vi "Main.vi"(9 "rSubPanel":refnum<vi>, 10 "模块定义":T1, 11 "Module Admin":refnum<class "Delacor_lib_QMH_Cloneable Module Admin.lvclass">) -> ()   [LabVIEW 2018, in "ModuleInterface.lvlib"]
doc: "This template is based off of the Queued Message Handler design pattern and the Queued Message Handler project template that ships with LabVIEW.\n\nThe main difference is that the queue is private to this module and communication between modules is performed via Broadcast and Request events.\n\nRequest events are wrapped in public API methods and are handled in the Event Handling Loop (EHL) of this VI. Any module can register for Broadcast events sent by this module. The EHL generates messages based on user interface actions.\n\nThe Message Handling Loop (MHL) processes messages generated by the EHL, or by other messages. The messages are string values, so new messages can be added easily to the Message Cases case structure in the MHL. Each message cluster can also provide an optional value for Message Data, which is a variant that can be converted to whatever message-specific data is required.\n_____\nBased on DQMH Project Template 7.0.1.1316."
uses:
  ModuleInterface.lvlib
  <vilib>/Delacor/Delacor QMH/Libraries/Cloneable Module Admin_class/Delacor_lib_QMH_Cloneable Module Admin.lvclass
  C:/Program Files (x86)/National Instruments/LabVIEW 2018/vi.lib/Delacor/Delacor QMH/Libraries/Module Admin_class/Delacor_lib_QMH_Module Admin.lvclass
  Buttons/FoldButton.ctl
  ModuleDefinition.ctl
  FunctionItem.ctl
  Module Data--cluster.ctl
  <vilib>/Delacor/Delacor QMH/Libraries/Message Queue_class/Delacor_lib_QMH_Message Queue.lvclass/Delacor_lib_QMH_Message Queue.ctl
  <vilib>/Delacor/Delacor QMH/Libraries/Cloneable Module Admin_class/Delacor_lib_QMH_Cloneable Module Admin.lvclass/Delacor_lib_QMH_Cloneable Module Admin.ctl
  Stop Argument--cluster.ctl
  <vilib>/Delacor/Delacor QMH/Libraries/Module Admin_class/Delacor_lib_QMH_Module Admin.lvclass/Delacor_lib_QMH_Module Admin.ctl
  Get Module Name Argument--cluster.ctl
  Get Module Name (Reply Payload)--cluster.ctl
  Get Module ID List Argument--cluster.ctl
  Get Module ID List (Reply Payload)--cluster.ctl
  Disable Item Argument--cluster.ctl
  Enable Item Argument--cluster.ctl
  <vilib>/Utility/miscctls.llb/LVPointTypeDef.ctl
  Clone Registration/Action--enum.ctl
  <vilib>/Delacor/Delacor QMH/Libraries/Message Queue_class/Delacor_lib_QMH_Enqueue Message (Single).vi
  <vilib>/Delacor/Delacor QMH/Libraries/Cloneable Module Admin_class/Delacor_lib_QMH_Get Module ID.vi
  <vilib>/Delacor/Delacor QMH/Libraries/Module Admin_class/Delacor_lib_QMH_Get External Launch.vi
  <vilib>/Delacor/Delacor QMH/Libraries/Message Queue_class/Delacor_lib_QMH_Message Queue.lvclass
  Clone Registration/Clone Registration.lvlib
panel:
  in  "界面单元":T4={"ModuleName"="", "FunctionList"=0, "展收按钮"=TRUE, "Spacer"=""}
  out "error out":errorcluster
  out "Status":string
  in  "Simulate EHL Error":bool
  in  "Simulate MHL Error":bool
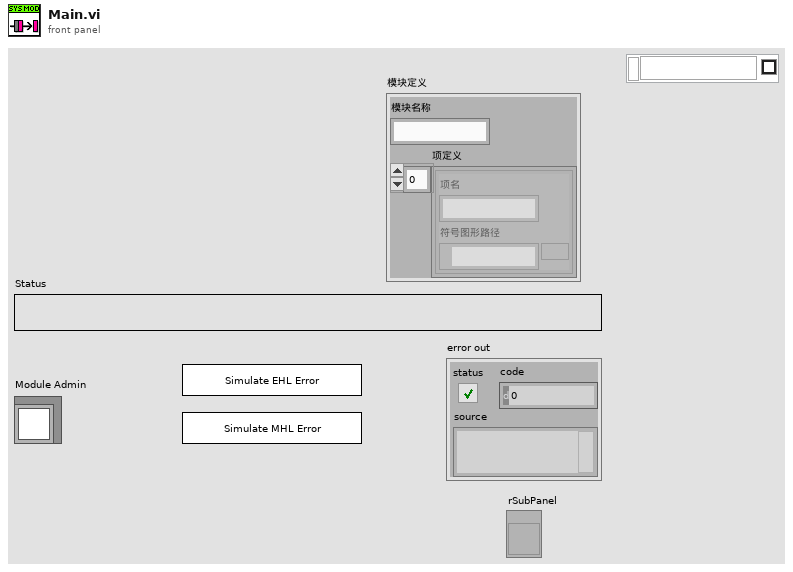
[diagram p1: front panel]
types:
  T1 = typedef "ModuleInterface.lvlib/ModuleDefinition.ctl" = cluster{"模块名称":string, "项定义":T2[]}
  T2 = typedef "ModuleInterface.lvlib/FunctionItem.ctl" = cluster{"项名":string, "符号图形路径":path}
  T3 = typedef "FoldButton.ctl" = bool
  T4 = cluster{"ModuleName":string, "FunctionList":i32, "展收按钮":T3, "Spacer":string}
  T5 = typedef "ModuleInterface.lvlib/Request Events--cluster.ctl" = cluster{"Stop Module":refnum<user-event>, "Show Panel":refnum<user-event>, "Hide Panel":refnum<user-event>, "Show Diagram":refnum<user-event>, "Get Module Execution Status":refnum<user-event>, "Get Module Name":refnum<user-event>, "Get Module ID List":refnum<user-event>, "Disable Item":refnum<user-event>, "Enable Item":refnum<user-event>}
  T6 = typedef "ModuleInterface.lvlib/Module Data--cluster.ctl" = cluster{"Status":string, "rSubPanel":refnum<vi>, "Disabled Items":string[]}
  T7 = enum32{"invalid lock state", "Not Locked", "Locked (No Password)", "Password-protected"}
  T8 = typedef "ModuleInterface.lvlib/Stop Argument--cluster.ctl" = cluster{"Module ID":i32, "Origin":string, "Exit via Stop Module Req?":bool, "Wait for Module to stop?":bool}
  T9 = typedef "ModuleInterface.lvlib/Get Module Name Argument--cluster.ctl" = cluster{"Module ID":i32, "Wait Notifier":refnum<notifier>, "wait for reply":bool}
  T10 = typedef "ModuleInterface.lvlib/Get Module ID List Argument--cluster.ctl" = cluster{"Module ID":i32, "Wait Notifier":refnum<notifier>, "wait for reply":bool}
  T11 = typedef "ModuleInterface.lvlib/Disable Item Argument--cluster.ctl" = cluster{"Module ID":i32, "Item Name":string}
  T12 = typedef "ModuleInterface.lvlib/Enable Item Argument--cluster.ctl" = cluster{"Module ID":i32, "Item Name":string}
  T13 = enum32{"Invalid", "Standard", "Closed", "Hidden", "Minimized", "Maximized"}
  T14 = typedef "LVPointTypeDef.ctl" = cluster{"Horizontal":i16, "Vertical":i16}
  T15 = typedef "ModuleInterface.lvlib/Get Module Name (Reply Payload)--cluster.ctl" = cluster{"Module ID":i32, "Module Name":string, "error":errorcluster}
  T16 = typedef "ModuleInterface.lvlib/Clone Registration.lvlib/Action--enum.ctl" = enum16{"Init", "Add Instance", "Remove Instance", "List Instances", "Is First?"}
  T17 = typedef "ModuleInterface.lvlib/Get Module ID List (Reply Payload)--cluster.ctl" = cluster{"Module ID":i32, "Module ID List":i32[], "error":errorcluster}
  T18 = typedef "LVRectTypeDef.ctl" = cluster{"Left":i16, "Top":i16, "Right":i16, "Bottom":i16}
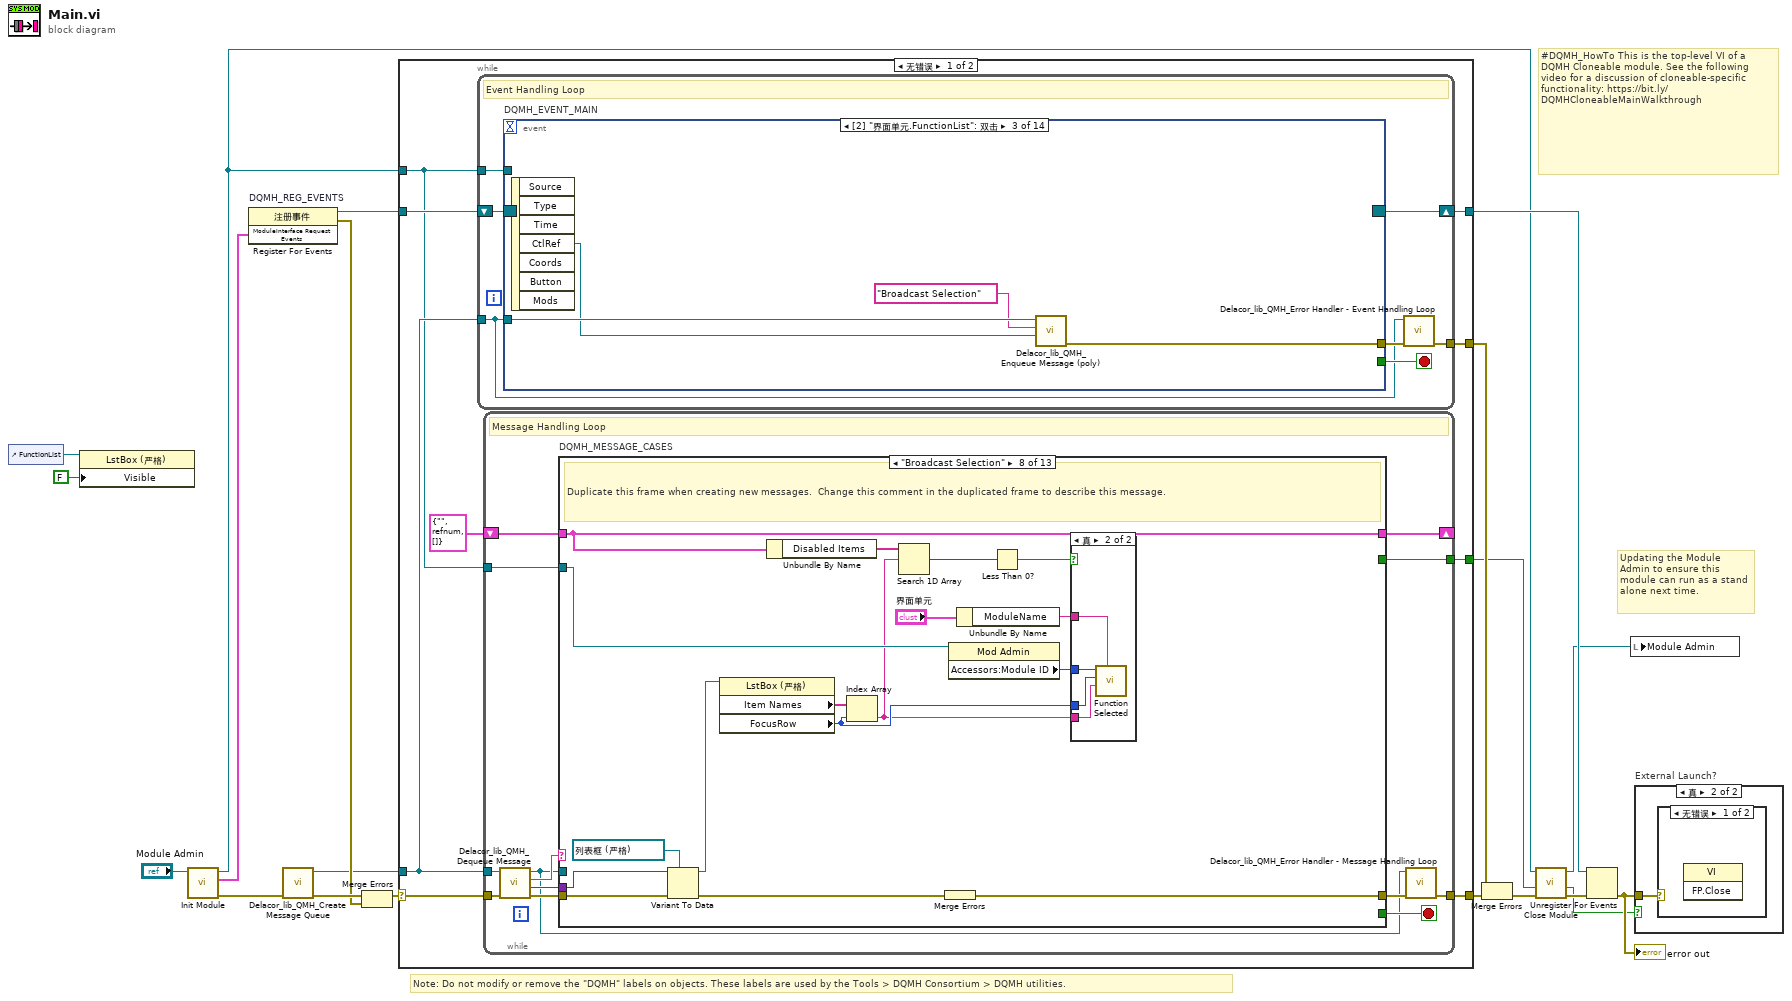
[diagram p0: block diagram]
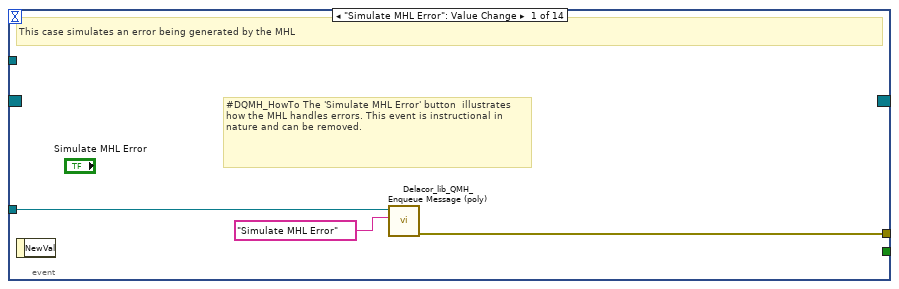
[diagram p2: hidden frame]
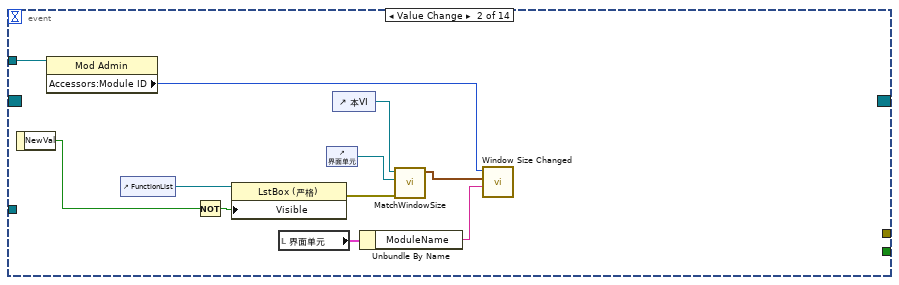
[diagram p3: hidden frame]
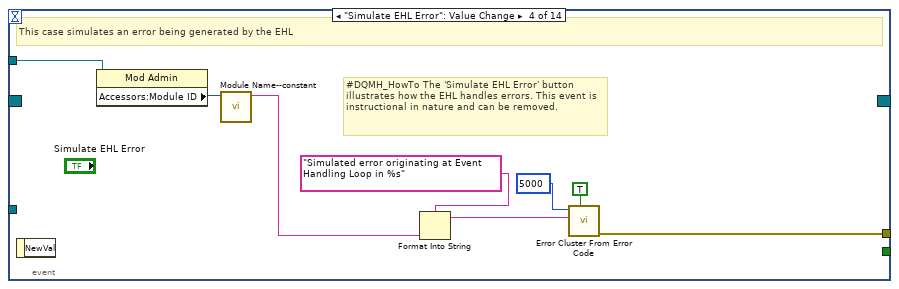
[diagram p4: hidden frame]
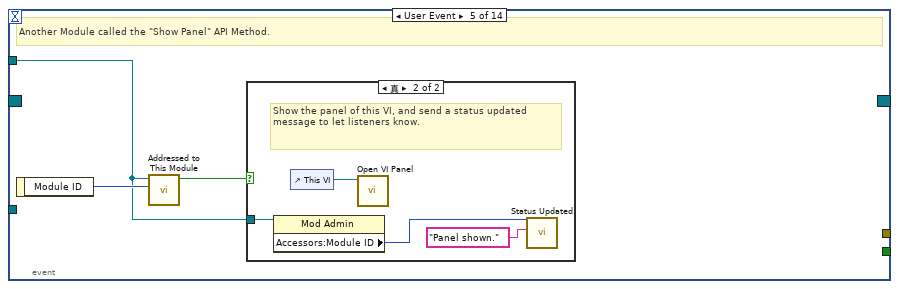
[diagram p5: hidden frame]
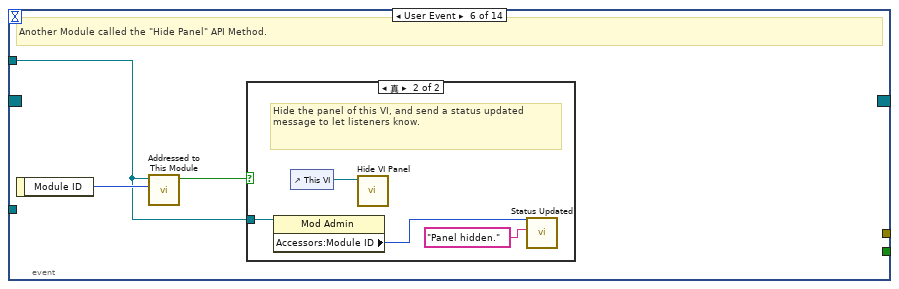
[diagram p7: hidden frame]
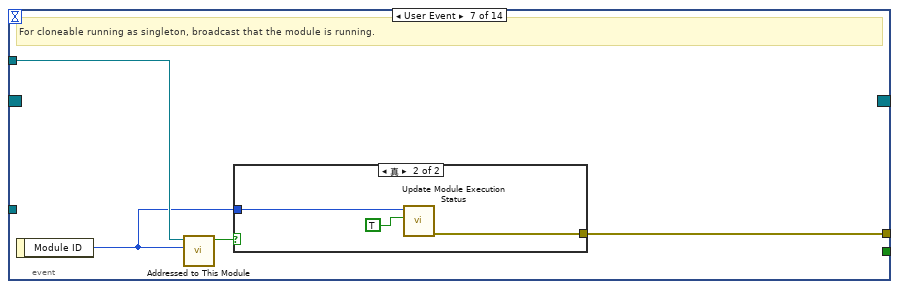
[diagram p9: hidden frame]
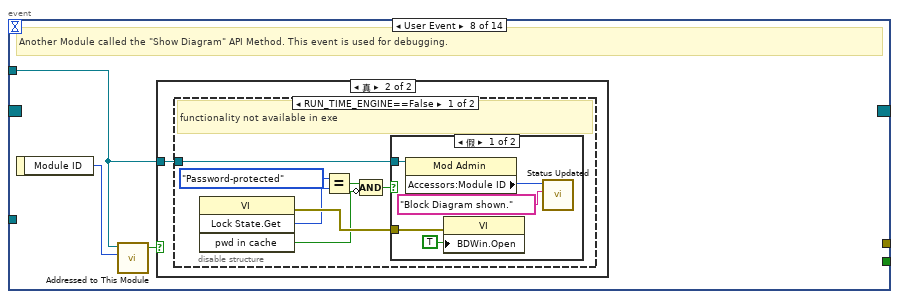
[diagram p11: hidden frame]
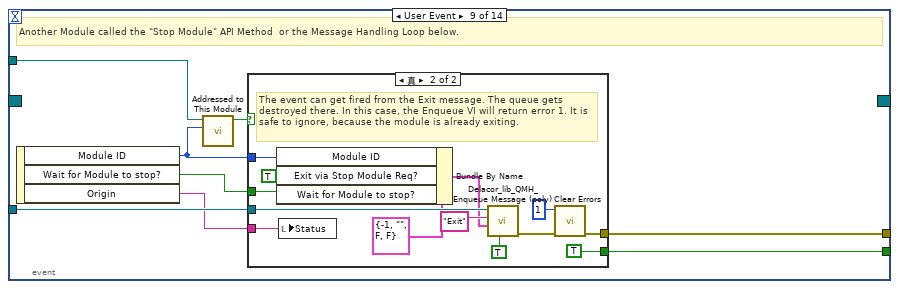
[diagram p15: hidden frame]
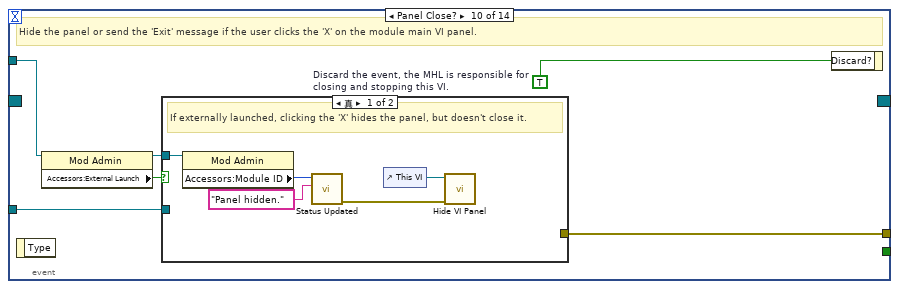
[diagram p17: hidden frame]
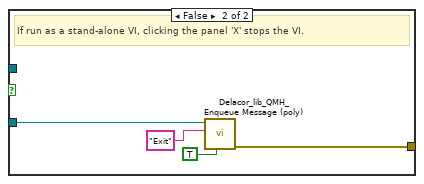
[diagram p18: hidden frame]
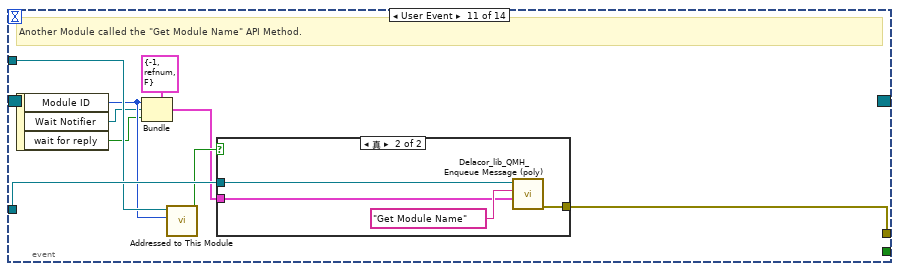
[diagram p19: hidden frame]
diagram:
  # "#DQMH_HowTo This is the top-level VI of a DQMH Cloneable module. See the following video for a discussion of cloneable-specific functionality: https://bit.ly/DQMHCloneableMainWalkthrough"
  # "Note: Do not modify or remove the \"DQMH\" labels on objects. These labels are used by the Tools > DQMH Consortium > DQMH utilities."
  # "Updating the Module Admin to ensure this module can run as a stand alone next time."
  n1 = control-ref of="FunctionList"() -> (w1:refnum<vi>)
  n2 = property class="LstBox (严格)"(reference=w1, "Visible"=FALSE ("可见")) -> ()  [unwired: 1 in, 2 out]
  n3 = call "Init Module.vi"("Cloneable Module Admin in"="Module Admin") -> ("error out"=w17:errorcluster, "ModuleInterface Request Events"=w9:T5, "Cloneable Module Admin out"=w6:refnum<class "Delacor_lib_QMH_Cloneable Module Admin.lvclass">)  [unwired: 8 in]
  n4 = register-events "DQMH_REG_EVENTS"(w9) -> (reference out=w10:refnum<event-registration>, error out=w12:errorcluster)  [unwired: 2 in]
  n5 = call <vilib>:"Delacor_lib_QMH_Create Message Queue.vi"("error in"=w17) -> ("error out"=w14:errorcluster, "Message Queue"=w8:refnum<class "Delacor_lib_QMH_Message Queue.lvclass">)  [unwired: 9 in]
  n6 = Merge Errors(w14, w12) -> (w13:errorcluster)
  n7 = case shown="无错误" w13 {
    selector: w13 -> [w27 w408]
    tunnel: [w29 w407] -> w18
    tunnel: [w26 w406] -> w11
    tunnel: w10 -> [w24 w406]
    tunnel: w8 -> [w23 w399]
    tunnel: [w28 _] -> w19
    tunnel: w6 -> [w22 w402]
    tunnel: [w21 _] -> w4
    frame No Error {
      n8 = while {
        tunnel: w23 -> [w30]
        shift-right: [w33] -> w26
        shift-left: w24 -> [w34]
        tunnel: [w35] -> w28
        tunnel: w22 -> [w31]
        stop <- w32 stop-if-true
        # "Event Handling Loop"
        n9 = event "DQMH_EVENT_MAIN" shown="[2] \"界面单元.FunctionList\": 双击" {
          selector: w34 -> [_ _ _ _ _ _ _ _ _ _ _ _ _ _]
          dyn-events: [_ _ _ _ _ _ _ _ _ _ _ _ _ _] -> w33
          timeout: _ -> [_ _ _ _ _ _ _ _ _ _ _ _ _ _]
          tunnel: [_ _ _ _ _ _ _ _ w103 _ _ _ _ _] -> w32
          tunnel: w30 -> [w38 _ w54 _ _ _ _ _ w106 w123 w144 w157 w169 w181]
          tunnel: [w39 _ w53 w62 _ _ w80 _ w107 w126 w136 w149 w162 w174] -> w36
          tunnel: w31 -> [_ w44 _ w61 w63 w70 w78 w84 w105 w124 w142 w155 w167 w179]
          event "Simulate MHL Error": Value Change {
            # "#DQMH_HowTo The 'Simulate MHL Error' button  illustrates how the MHL handles errors. This event is instructional in nature and can be removed."
            # "This case simulates an error being generated by the MHL"
            n10 = event-data() -> ()  [unwired: 1 in, 1 out]
            n11 = call-poly <vilib>:"Delacor_lib_QMH_Enqueue Message (poly).vi"("Message"="Simulate MHL Error", "Message Queue in"=w38) -> ("error out"=w39:errorcluster)  [unwired: 8 in, 1 out]
          }
          event Value Change {
            n12 = event-data() -> ("NewVal"=w49:T3)  [unwired: 1 in]
            n13 = property on="Property Node" class="Mod Admin"(reference=w44) -> ("Accessors:Module ID"=w42:i32)  [unwired: 1 in, 2 out]
            n14 = control-ref of="FunctionList"() -> (w50:refnum<vi>)
            n15 = Not(x=w49) -> (.not. x?=w48:T3)
            n16 = property class="LstBox (严格)"(reference=w50, "Visible"=w48) -> (error out=w46:errorcluster)  [unwired: 1 in, 1 out]
            n17 = local read "界面单元"() -> (w41:T4)
            n18 = control-ref of="界面单元"() -> (w47:refnum<vi>)
            n19 = control-ref of="本VI"() -> (w45:refnum<vi>)
            n20 = Unbundle By Name(w41) -> ("ModuleName"=w40:string)
            n21 = call "MatchWindowSize.vi"("错误输入（无错误）"=w46, "界面单元"=w47, "VI输入"=w45) -> ("窗口边界"=w43:T18)  [unwired: 7 in, 1 out]
            n22 = call "Window Size Changed.vi"("Module Name"=w40, "窗口边界"=w43, "Module ID"=w42) -> ()  [unwired: 8 in, 1 out]
          }
          event "界面单元.FunctionList": Double Click {
            n23 = event-data() -> ("CtlRef"=w52:refnum<vi>)  [unwired: 1 in, 6 out]
            n24 = call-poly <vilib>:"Delacor_lib_QMH_Enqueue Message (poly).vi"("Message Data"=w52, "Message"="Broadcast Selection", "Message Queue in"=w54) -> ("error out"=w53:errorcluster)  [unwired: 7 in, 1 out]
          }
          event "Simulate EHL Error": Value Change {
            # "#DQMH_HowTo The 'Simulate EHL Error' button  illustrates how the EHL handles errors. This event is instructional in nature and can be removed."
            # "This case simulates an error being generated by the EHL"
            n25 = event-data() -> ()  [unwired: 1 in, 1 out]
            n26 = property on="Property Node" class="Mod Admin"(reference=w61) -> ("Accessors:Module ID"=w60:i32)  [unwired: 1 in, 2 out]
            n27 = call "Module Name--constant.vi"("Module ID"=w60) -> ("Module Name"=w55:string)  [unwired: 10 in]
            n28 = Format Into String(format string="Simulated error originating at Event Handling Loop in %s", w55) -> (resulting string=w58:string)  [unwired: 2 in, 1 out]
            n29 = call <vilib>:"Error Cluster From Error Code.vi"("show call chain? (False)"=TRUE, "error message (\"\")"=w58, "error code (0)"=5000) -> ("error out"=w62:errorcluster)  [unwired: 6 in]
          }
          event User Event {
            # "Another Module called the \"Show Panel\" API Method."
            n30 = event-data() -> ("Module ID"=w64:i32)  [unwired: 1 in]
            n31 = call "Addressed to This Module.vi"("Module ID from Argument"=w64, "Module Admin"=w63) -> ("Addressed to this instance?"=w65:bool)  [unwired: 8 in, 1 out]
            n32 = case shown="真" w65 {
              tunnel: w63 -> [_ w67]
              frame False {
              }
              frame True {
                # "Show the panel of this VI, and send a status updated message to let listeners know."
                n33 = property on="Property Node" class="Mod Admin"(reference=w67) -> ("Accessors:Module ID"=w66:i32)  [unwired: 1 in, 2 out]
                n34 = control-ref of="This VI"() -> (w69:refnum<vi>)
                n35 = call "Open VI Panel.vi"("VI"=w69) -> ()  [unwired: 10 in, 1 out]
                n36 = call "Status Updated.vi"("Status"="Panel shown." ("format string"), "Module ID"=w66) -> ()  [unwired: 9 in, 1 out]
              }
            }
          }
          event User Event {
            # "Another Module called the \"Hide Panel\" API Method."
            n37 = event-data() -> ("Module ID"=w71:i32)  [unwired: 1 in]
            n38 = call "Addressed to This Module.vi"("Module ID from Argument"=w71, "Module Admin"=w70) -> ("Addressed to this instance?"=w72:bool)  [unwired: 8 in, 1 out]
            n39 = case shown="真" w72 {
              tunnel: w70 -> [_ w74]
              frame False {
              }
              frame True {
                # "Hide the panel of this VI, and send a status updated message to let listeners know."
                n40 = property on="Property Node" class="Mod Admin"(reference=w74) -> ("Accessors:Module ID"=w73:i32)  [unwired: 1 in, 2 out]
                n41 = control-ref of="This VI"() -> (w76:refnum<vi>)
                n42 = call "Hide VI Panel.vi"("VI"=w76) -> ()  [unwired: 10 in, 1 out]
                n43 = call "Status Updated.vi"("Status"="Panel hidden." ("format string"), "Module ID"=w73) -> ()  [unwired: 9 in, 1 out]
              }
            }
          }
          event User Event {
            # "For cloneable running as singleton, broadcast that the module is running."
            n44 = event-data() -> ("Module ID"=w77:i32)  [unwired: 1 in]
            n45 = call "Addressed to This Module.vi"("Module ID from Argument"=w77, "Module Admin"=w78) -> ("Addressed to this instance?"=w79:bool)  [unwired: 8 in, 1 out]
            n46 = case shown="真" w79 {
              tunnel: [_ w83] -> w80
              tunnel: w77 -> [_ w82]
              frame False {
              }
              frame True {
                n47 = call "Update Module Execution Status.vi"("Running?"=TRUE, "Module ID"=w82) -> ("error out"=w83:errorcluster)  [unwired: 9 in]
              }
            }
          }
          event User Event {
            # "Another Module called the \"Show Diagram\" API Method. This event is used for debugging."
            n48 = event-data() -> ("Module ID"=w85:i32)  [unwired: 1 in]
            n49 = call "Addressed to This Module.vi"("Module ID from Argument"=w85, "Module Admin"=w84) -> ("Addressed to this instance?"=w86:bool)  [unwired: 8 in, 1 out]
            n50 = case shown="真" w86 {
              tunnel: w84 -> [_ w87]
              frame False {
              }
              frame True {
                n51 = disable-structure shown="RUN_TIME_ENGINE==False" {
                  disable-tunnel: w87 -> [w88 _]
                  frame condition #0 (active) {
                    # "functionality not available in exe"
                    n52 = invoke on="Invoke Node" class="VI" method="Lock State.Get"() -> (error out=w94:errorcluster, "Get Lock State"=w93:T7, "pwd in cache"=w90:bool)  [unwired: 4 in, 1 out]
                    n53 = Equal?(x=T7."Password-protected", y=w93) -> (x = y?=w91:bool)
                    n54 = Compound Arithmetic op=AND(w91, invert w90) -> (w89:bool)
                    n55 = case shown="假" w89 {
                      tunnel: w94 -> [w99 _]
                      tunnel: w88 -> [w96 _]
                      frame False {
                        n56 = property on="Property Node" class="Mod Admin"(reference=w96) -> ("Accessors:Module ID"=w95:i32)  [unwired: 1 in, 2 out]
                        n57 = property on="Property Node" class="VI"(error in=w99, "BDWin.Open"=TRUE ("Block Diagram Window:Open")) -> ()  [unwired: 1 in, 2 out]
                        n58 = call "Status Updated.vi"("Status"="Block Diagram shown." ("format string"), "Module ID"=w95) -> ()  [unwired: 9 in, 1 out]
                      }
                      frame True {
                        # "Password-protected VI, and the password is not in the cache. Do not show the diagram."
                      }
                    }
                  }
                  frame condition #1 {
                  }
                }
              }
            }
          }
          event User Event {
            # "Another Module called the \"Stop Module\" API Method  or the Message Handling Loop below."
            n59 = event-data() -> ("Module ID"=w101:i32, "Wait for Module to stop?"=w102:bool, "Origin"=w100:string)  [unwired: 1 in]
            n60 = call "Addressed to This Module.vi"("Module ID from Argument"=w101, "Module Admin"=w105) -> ("Addressed to this instance?"=w104:bool)  [unwired: 8 in, 1 out]
            n61 = case shown="真" w104 {
              tunnel: [_ w119] -> w107
              tunnel: w106 -> [_ w115]
              tunnel: [_ TRUE] -> w103
              tunnel: w102 -> [_ w110]
              tunnel: w101 -> [_ w112]
              tunnel: w100 -> [_ w108]
              frame False {
              }
              frame True {
                # "The event can get fired from the Exit message. The queue gets destroyed there. In this case, the Enqueue VI will return error 1. It is safe to ignore, because the module is already exiting."
                n62 = Bundle By Name(cluster=T8 {"Module ID"=-1, "Origin"="", "Exit via Stop Module Req?"=FALSE, "Wait for Module to stop?"=FALSE} ("Stop Argument"), "Module ID"=w112, "Exit via Stop Module Req?"=TRUE, "Wait for Module to stop?"=w110) -> (w109:T8)
                n63 = local write "Status"(w108) -> ()
                n64 = call-poly <vilib>:"Delacor_lib_QMH_Enqueue Message (poly).vi"("Priority Message? (F)"=TRUE, "Message Data"=w109, "Message"="Exit", "Message Queue in"=w115) -> ("error out"=w120:errorcluster)  [unwired: 6 in, 1 out]
                n65 = call <vilib>:"Clear Errors.vi"("error in (no error)"=w120, "specific error code to clear (0: all)"=1) -> ("error out"=w119:errorcluster)  [unwired: 4 in, 1 out]
              }
            }
          }
          event Panel Close? {
            w125 = TRUE  # Discard the event, the MHL is responsible for closing and stopping this VI.
            # "Hide the panel or send the 'Exit' message if the user clicks the 'X' on the module main VI panel."
            n66 = event-data() -> ()  [unwired: 1 in, 1 out]
            n67 = property on="Property Node" class="Mod Admin"(reference=w124) -> (reference out=w121:refnum<class "Delacor_lib_QMH_Cloneable Module Admin.lvclass">, "Accessors:External Launch"=w122:bool)  [unwired: 1 in, 1 out]
            n68 = case shown="真" w122 {
              tunnel: w123 -> [_ w134]
              tunnel: [_ w135] -> w126
              tunnel: w121 -> [w129 _]
              frame True {
                # "If externally launched, clicking the 'X' hides the panel, but doesn't close it."
                n69 = property on="Property Node" class="Mod Admin"(reference=w129) -> ("Accessors:Module ID"=w128:i32)  [unwired: 1 in, 2 out]
                n70 = call "Status Updated.vi"("Status"="Panel hidden." ("format string"), "Module ID"=w128) -> ("error out"=w127:errorcluster)  [unwired: 9 in]
                n71 = control-ref of="This VI"() -> (w131:refnum<vi>)
                n72 = call "Hide VI Panel.vi"("error in"=w127, "VI"=w131) -> ()  [unwired: 9 in, 1 out]
              }
              frame False {
                # "If run as a stand-alone VI, clicking the panel 'X' stops the VI."
                n73 = call-poly <vilib>:"Delacor_lib_QMH_Enqueue Message (poly).vi"("Priority Message? (F)"=TRUE, "Message"="Exit", "Message Queue in"=w134) -> ("error out"=w135:errorcluster)  [unwired: 7 in, 1 out]
              }
            }
            n74 = event-data ("Event Filter Node")("Discard?"=w125) -> ()  [unwired: 1 in, 1 out]
          }
          event User Event {
            # "Another Module called the \"Get Module Name\" API Method."
            n75 = event-data() -> ("Module ID"=w139:i32, "Wait Notifier"=w138:refnum<notifier>, "wait for reply"=w137:bool)  [unwired: 1 in]
            n76 = Bundle(cluster=T9 {"Module ID"=-1, "Wait Notifier"=refnum, "wait for reply"=FALSE} ("Get Module Name Argument"), "Module ID"=w139, "Wait Notifier"=w138, "wait for reply"=w137) -> (w140:T9)
            n77 = call "Addressed to This Module.vi"("Module ID from Argument"=w139, "Module Admin"=w142) -> ("Addressed to this instance?"=w143:bool)  [unwired: 8 in, 1 out]
            n78 = case "条件结构" shown="真" w143 {
              tunnel: w144 -> [_ w148]
              tunnel: w140 -> [_ w146]
              tunnel: [_ w145] -> w136
              frame False {
              }
              frame True {
                n79 = call-poly <vilib>:"Delacor_lib_QMH_Enqueue Message (poly).vi"("Message Data"=w146, "Message"="Get Module Name", "Message Queue in"=w148) -> ("error out"=w145:errorcluster)  [unwired: 7 in, 1 out]
              }
            }
          }
          event User Event {
            # "Another Module called the \"Get Module ID List\" API Method."
            n80 = event-data() -> ("Module ID"=w152:i32, "Wait Notifier"=w151:refnum<notifier>, "wait for reply"=w150:bool)  [unwired: 1 in]
            n81 = Bundle(cluster=T10 {"Module ID"=-1, "Wait Notifier"=refnum, "wait for reply"=FALSE} ("Get Module ID List Argument"), "Module ID"=w152, "Wait Notifier"=w151, "wait for reply"=w150) -> (w153:T10)
            n82 = call "Addressed to This Module.vi"("Module ID from Argument"=w152, "Module Admin"=w155) -> ("Addressed to this instance?"=w156:bool)  [unwired: 8 in, 1 out]
            n83 = case "条件结构" shown="真" w156 {
              tunnel: w157 -> [_ w161]
              tunnel: w153 -> [_ w159]
              tunnel: [_ w158] -> w149
              frame False {
              }
              frame True {
                n84 = call-poly <vilib>:"Delacor_lib_QMH_Enqueue Message (poly).vi"("Message Data"=w159, "Message"="Get Module ID List", "Message Queue in"=w161) -> ("error out"=w158:errorcluster)  [unwired: 7 in, 1 out]
              }
            }
          }
          event User Event {
            # "Another Module called the \"Disable Item\" API Method."
            n85 = event-data() -> ("Module ID"=w164:i32, "Item Name"=w163:string)  [unwired: 1 in]
            n86 = Bundle(cluster=T11 {"Module ID"=-1, "Item Name"=""} ("Disable Item Argument"), "Module ID"=w164, "Item Name"=w163) -> (w165:T11)
            n87 = call "Addressed to This Module.vi"("Module ID from Argument"=w164, "Module Admin"=w167) -> ("Addressed to this instance?"=w168:bool)  [unwired: 8 in, 1 out]
            n88 = case "条件结构" shown="真" w168 {
              tunnel: w169 -> [_ w173]
              tunnel: w165 -> [_ w171]
              tunnel: [_ w170] -> w162
              frame False {
              }
              frame True {
                n89 = call-poly <vilib>:"Delacor_lib_QMH_Enqueue Message (poly).vi"("Message Data"=w171, "Message"="Disable Item", "Message Queue in"=w173) -> ("error out"=w170:errorcluster)  [unwired: 7 in, 1 out]
              }
            }
          }
          event User Event {
            # "Another Module called the \"Enable Item\" API Method."
            n90 = event-data() -> ("Module ID"=w176:i32, "Item Name"=w175:string)  [unwired: 1 in]
            n91 = Bundle(cluster=T12 {"Module ID"=-1, "Item Name"=""} ("Enable Item Argument"), "Module ID"=w176, "Item Name"=w175) -> (w177:T12)
            n92 = call "Addressed to This Module.vi"("Module ID from Argument"=w176, "Module Admin"=w179) -> ("Addressed to this instance?"=w180:bool)  [unwired: 8 in, 1 out]
            n93 = case "条件结构" shown="真" w180 {
              tunnel: w181 -> [_ w185]
              tunnel: w177 -> [_ w183]
              tunnel: [_ w182] -> w174
              frame False {
              }
              frame True {
                n94 = call-poly <vilib>:"Delacor_lib_QMH_Enqueue Message (poly).vi"("Message Data"=w183, "Message"="Enable Item", "Message Queue in"=w185) -> ("error out"=w182:errorcluster)  [unwired: 7 in, 1 out]
              }
            }
          }
        }
        n95 = call-dynamic "Delacor_lib_QMH_Error Handler - Event Handling Loop.vi"("error in"=w36, "Message Queue in"=w30) -> ("dup error in"=w35:errorcluster)  [unwired: 8 in, 1 out]
      }
      n96 = while {
        tunnel: w23 -> [w186]
        shift-right: [w193] -> _
        shift-left: T6 {"Status"="", "rSubPanel"=refnum, "Disabled Items"=[]} ("Data Cluster") -> [w194]
        tunnel: w27 -> [w197]
        tunnel: [w195] -> w29
        tunnel: w22 -> [w188]
        tunnel: [w187] -> w21
        stop <- w192 stop-if-true
        # "Message Handling Loop"
        n97 = call-dynamic "Delacor_lib_QMH_Dequeue Message.vi"("error in"=w197, "Message Queue in"=w186) -> ("error out"=w196:errorcluster, "Message Data"=w190:variant, "Message"=w191:string, "Message Queue out"=w189:refnum<class "Delacor_lib_QMH_Message Queue.lvclass">)  [unwired: 6 in]
        n98 = case "DQMH_MESSAGE_CASES" shown="\"Broadcast Selection\"" w191 {
          selector: w191 -> [_ _ _ _ _ _ _ _ _ _ _ _ w388]
          tunnel: w189 -> [_ _ _ _ _ _ _ _ _ w341 _ w380 _]
          tunnel: w196 -> [w230 w232 w247 w263 w280 w302 w315 w332 w338 w350 w367 w386 w397]
          tunnel: [w229 w232 w237 w261 w279 w301 w314 w331 w338 w346 w366 w381 w398] -> w198
          tunnel: w194 -> [w227 w231 w246 w262 w269 w292 w313 w320 w337 w345 w364 w369 w395]
          tunnel: [w226 w231 w246 w262 w267 w289 w313 w320 w337 w345 w364 w369 w395] -> w193
          tunnel: [_ _ _ _ _ _ _ _ _ _ _ w379 _] -> w192
          tunnel: w190 -> [_ _ w244 w260 w278 w300 _ w329 _ w344 _ w377 _]
          tunnel: w188 -> [w223 _ w235 w252 _ _ _ w322 _ w343 w362 w372 w394]
          tunnel: [_ _ _ _ _ _ _ _ _ _ _ w375 _] -> w187
          frame "Initialize" {
            w221 = "Initial Message" ("Initial Message")
            # "Initialize - Any operation that needs to be done before the module can receive messages. Synchronize Caller Events.vi will inform Start Module.vi that the module has launched and is ready to receive messages. Module Did Init.vi will broadcast that the module initialized."
            n99 = call "Synchronize Caller Events.vi"("error in"=w230, "Module Admin"=w223) -> ("error out"=w212:errorcluster, "Module Admin out"=w222:refnum<class "Delacor_lib_QMH_Cloneable Module Admin.lvclass">)  [unwired: 8 in]
            n100 = property on="Property Node" class="Mod Admin"(reference=w222) -> ("Accessors:Module ID"=w205:i32)  [unwired: 1 in, 2 out]
            n101 = call "Module Name--constant.vi"("Module ID"=w205) -> ("Module Name"=w228:string)  [unwired: 10 in]
            n102 = control-ref of="FunctionList"() -> (w217:refnum<vi>)
            n103 = control-ref of="ModuleName"() -> (w214:refnum<vi>)
            n104 = property on="Property Node" class="VI"("Front Panel.Title"=w228) -> (reference out=w209:refnum<vi>, error out=w211:errorcluster)  [unwired: 2 in]
            n105 = invoke on="Invoke Node" class="VI" method="FP.Open"(reference=w209, error in=w211, "State"=T13."Standard") -> (reference out=w208:refnum<vi>, error out=w210:errorcluster)  [unwired: 2 in, 3 out]
            n106 = Bundle By Name(cluster=w227, "Status"=w221, "rSubPanel"="rSubPanel", "Disabled Items"=string[] []) -> (w226:T6)
            n107 = call "InitializeFunctionList.vi"("错误输入（无错误）"=w212, "模块定义"="模块定义", "rModuleName"=w214, "rFunctionList"=w217) -> ("错误输出"=w216:errorcluster)  [unwired: 7 in]
            n108 = invoke on="Invoke Node" class="VI" method="FP.Center"(reference=w208, error in=w210) -> (reference out=w206:refnum<vi>)  [unwired: 1 in, 2 out]
            n109 = control-ref of="本VI"() -> (w219:refnum<vi>)
            n110 = control-ref of="界面单元"() -> (w218:refnum<vi>)
            n111 = local read "界面单元"() -> (w203:T4)
            n112 = call "MatchWindowSize.vi"("错误输入（无错误）"=w216, "界面单元"=w218, "VI输入"=w219) -> ("错误输出"=w213:errorcluster, "窗口边界"=w204:T18)  [unwired: 7 in]
            n113 = Unbundle By Name(w203) -> ("ModuleName"=w202:string)
            n114 = property on="Pane" class="Pane"("Origin"=T14 {"Horizontal"=0, "Vertical"=0}) -> ()  [unwired: 2 in, 2 out]
            n115 = call "Insert SubPanel.vi"("VI Ref"=w206, "Subpanel Ref"="rSubPanel") -> ("error out"=w201:errorcluster)  [unwired: 9 in]
            n116 = call "Module Name--constant.vi"("Module ID"=w205) -> ("Module Name"=w224:string)  [unwired: 10 in]
            n117 = call <vilib>:"Clear Errors.vi"("error in (no error)"=w201) -> ()  [unwired: 5 in, 2 out]
            n118 = call "Module Did Init.vi"("error in"=w213, "Initialized?"=TRUE, "Origin"=w224, "Module ID"=w205) -> ("error out"=w229:errorcluster)  [unwired: 7 in]
            n119 = call "Window Size Changed.vi"("Module Name"=w202, "窗口边界"=w204, "Module ID"=w205) -> ()  [unwired: 8 in, 1 out]
            "Status" <- w221
          }
          frame "---Module Specific---" {
            # "Separator -- The following cases handle messages specific to this Module."
          }
          frame "Get Module Name" {
            n120 = property class="Mod Admin"(reference=w235) -> ("Accessors:Module ID"=w236:i32)  [unwired: 1 in, 2 out]
            n121 = Variant To Data(error in=w247, type=T9 {"Module ID"=-1, "Wait Notifier"=refnum, "wait for reply"=FALSE} ("Get Module Name Argument"), Variant=w244) -> (data=w242:T9, error out=w245:errorcluster)
            n122 = Unbundle By Name(w242) -> ("Wait Notifier"=w241:refnum<notifier>, "wait for reply"=w240:bool)  [unwired: 1 out]
            n123 = local read "界面单元"() -> (w234:T4)
            n124 = Unbundle By Name(w234) -> ("ModuleName"=w233:string)
            n125 = Bundle By Name(cluster=T15 {"Module ID"=-1, "Module Name"="", "error"={"status"=FALSE, "code"=0, "source"=""}} ("Get Module Name (Reply Payload)"), "Module ID"=w236, "Module Name"=w233) -> (w239:T15)
            n126 = Merge Errors(w245) -> (w237:errorcluster)
            n127 = case "DQMH_FIRE_NOTIFIER" shown="真" w240 {
              tunnel: w241 -> [_ w249]
              tunnel: w239 -> [_ w248]
              frame False {
              }
              frame True {
                n128 = Send Notification(notification=w248, notifier=w249) -> ()  [unwired: 1 in, 2 out]
              }
            }
          }
          frame "Get Module ID List" {
            n129 = property class="Mod Admin"(reference=w252) -> ("Accessors:Module ID"=w253:i32)  [unwired: 1 in, 2 out]
            n130 = Variant To Data(error in=w263, type=T10 {"Module ID"=-1, "Wait Notifier"=refnum, "wait for reply"=FALSE} ("Get Module ID List Argument"), Variant=w260) -> (data=w258:T10, error out=w261:errorcluster)
            n131 = Unbundle By Name(w258) -> ("Wait Notifier"=w257:refnum<notifier>, "wait for reply"=w256:bool)  [unwired: 1 out]
            n132 = call "Clone Registration AE.vi"("Action"=Action--enum."List Instances") -> ("Module IDs"=w250:i32[])  [unwired: 6 in, 8 out]
            n133 = Bundle By Name(cluster=T17 {"Module ID"=-1, "Module ID List"=[], "error"={"status"=FALSE, "code"=0, "source"=""}} ("Get Module ID List (Reply Payload)"), "Module ID"=w253, "Module ID List"=w250) -> (w255:T17)
            n134 = case "DQMH_FIRE_NOTIFIER" shown="真" w256 {
              tunnel: w257 -> [_ w265]
              tunnel: w255 -> [_ w264]
              frame False {
              }
              frame True {
                n135 = Send Notification(notification=w264, notifier=w265) -> ()  [unwired: 1 in, 2 out]
              }
            }
          }
          frame "Disable Item" {
            n136 = Variant To Data(error in=w280, type=T11 {"Module ID"=-1, "Item Name"=""} ("Disable Item Argument"), Variant=w278) -> (data=w276:T11, error out=w279:errorcluster)
            n137 = control-ref of="FunctionList"() -> (w275:refnum<vi>)
            n138 = property class="LstBox (严格)"(reference=w275) -> (reference out=w271:refnum<vi>, "Item Names"=w274:string[])  [unwired: 1 in, 1 out]
            n139 = Unbundle By Name(w276) -> ("Item Name"=w270:string)
            n140 = Unbundle By Name(w269) -> ("Disabled Items"=w266:string[])
            n141 = Search 1D Array(1D array=w274, element=w270) -> (index of element=w272:i32)  [unwired: 1 in]
            n142 = Greater Or Equal To 0?(x=w272) -> (x >= 0?=w273:bool)
            n143 = case shown="真" w273 {
              tunnel: w272 -> [_ w286]
              tunnel: w271 -> [_ w287]
              tunnel: w270 -> [_ w284]
              tunnel: [w281 w283] -> w268
              tunnel: w266 -> [w281 w282]
              frame False {
              }
              frame True {
                n144 = property class="LstBox (严格)"(reference=w287, "Active Row"=w286, "CellFontColor"=u32 9868950 ("活动行:单元格字体:颜色")) -> ()  [unwired: 1 in, 2 out]
                n145 = Build Array (concatenate)(w282, w284) -> (w283:string[])
              }
            }
            n146 = Bundle By Name(cluster=w269, "Disabled Items"=w268) -> (w267:T6)
          }
          frame "Enable Item" {
            n147 = Variant To Data(error in=w302, type=T12 {"Module ID"=-1, "Item Name"=""} ("Enable Item Argument"), Variant=w300) -> (data=w298:T12, error out=w301:errorcluster)
            n148 = control-ref of="FunctionList"() -> (w297:refnum<vi>)
            n149 = Unbundle By Name(w298) -> ("Item Name"=w290:string)
            n150 = property class="LstBox (严格)"(reference=w297) -> (reference out=w293:refnum<vi>, "Item Names"=w296:string[])  [unwired: 1 in, 1 out]
            n151 = Unbundle By Name(w292) -> ("Disabled Items"=w291:string[])
            n152 = Search 1D Array(1D array=w296, element=w290) -> (index of element=w294:i32)  [unwired: 1 in]
            n153 = Greater Or Equal To 0?(x=w294) -> (x >= 0?=w295:bool)
            n154 = case shown="真" w295 {
              tunnel: w294 -> [_ w308]
              tunnel: w293 -> [_ w309]
              tunnel: w291 -> [w303 w306]
              tunnel: w290 -> [_ w305]
              tunnel: [w303 w304] -> w288
              frame False {
              }
              frame True {
                n155 = property class="LstBox (严格)"(reference=w309, "Active Row"=w308, "CellFontColor"=u32 7 ("活动行:单元格字体:颜色")) -> ()  [unwired: 1 in, 2 out]
                n156 = for {
                  tunnel: w306 -> [w311] mode=indexing
                  tunnel: w305 -> [w312]
                  tunnel: [w311] -> w304 mode=indexing if=w310
                  n157 = Not Equal?(x=w311, y=w312) -> (x != y?=w310:bool)
                }
              }
            }
            n158 = Bundle By Name(cluster=w292, "Disabled Items"=w288) -> (w289:T6)
          }
          frame "---Copy This Frame---" {
            # "Duplicate this frame when creating new messages.  Change this comment in the duplicated frame to describe this message."
            n159 = Merge Errors(w315) -> (w314:errorcluster)
          }
          frame "Broadcast Selection" {
            # "Duplicate this frame when creating new messages.  Change this comment in the duplicated frame to describe this message."
            n160 = Variant To Data(error in=w332, type=refnum<vi> refnum ("控件引用"), Variant=w329) -> (data=w321:refnum<vi>, error out=w330:errorcluster)
            n161 = property class="LstBox (严格)"(reference=w321) -> ("Item Names"=w326:string[], "FocusRow"=w327:i32)  [unwired: 1 in, 2 out]
            n162 = Unbundle By Name(w320) -> ("Disabled Items"=w319:string[])
            n163 = Index Array(array=w326, index=w327) -> (element=w318:string)
            n164 = Search 1D Array(1D array=w319, element=w318) -> (index of element=w317:i32)  [unwired: 1 in]
            n165 = Merge Errors(w330) -> (w331:errorcluster)
            n166 = property on="Property Node" class="Mod Admin"(reference=w322) -> ("Accessors:Module ID"=w323:i32)  [unwired: 1 in, 2 out]
            n167 = Unbundle By Name("界面单元") -> ("ModuleName"=w325:string)
            n168 = Less Than 0?(x=w317) -> (x < 0?=w316:bool)
            n169 = case shown="真" w316 {
              tunnel: w318 -> [_ w336]
              tunnel: w327 -> [_ w335]
              tunnel: w325 -> [_ w334]
              tunnel: w323 -> [_ w333]
              frame False {
              }
              frame True {
                n170 = call "Function Selected.vi"("Module Name"=w334, "Item Name"=w336, "ItemIndex"=w335, "Module ID"=w333) -> ()  [unwired: 7 in, 1 out]
              }
            }
          }
          frame "---Exit and Error Handling---" {
            # "Separator - the following cases handle errors and exit messages."
          }
          frame "Error" {
            # "#CodeRecommended - If the module is running in standalone mode (External Launch = FALSE), this code will pop up an error dialog and call the 'Exit' message if an error occurs. Add more fine-grained error management here."
            # "Error - Check the error message data and respond accordingly. This message is sent by the \"Error Handler\" VIs at the end of each loop in this application."
            n171 = property on="Property Node" class="Mod Admin"(reference=w343) -> ("Accessors:External Launch"=w342:bool, "Accessors:Module ID"=w340:i32)  [unwired: 1 in, 2 out]
            n172 = Variant To Data(error in=w350, type=errorcluster {"status"=FALSE, "code"=0, "source"=""} ("error constant"), Variant=w344) -> (data=w339:errorcluster, error out=w348:errorcluster)
            n173 = local write "error out"(w339) -> ()
            n174 = call "Error Reported.vi"("Error"=w339, "Module ID"=w340) -> ()  [unwired: 9 in, 1 out]
            n175 = case shown="假" w342 {
              tunnel: [w355 _] -> w347
              tunnel: w341 -> [w353 _]
              tunnel: w339 -> [w354 _]
              frame False {
                n176 = disable-structure shown="Default" {
                  disable-tunnel: w354 -> [w356 _]
                  frame condition #0 (active) {
                    # "If the module is running standalone, then pop up an error dialog and call the \"Exit\" message."
                    n177 = call <vilib>:"Simple Error Handler.vi"("error in (no error)"=w356) -> ()  [unwired: 4 in, 5 out]
                  }
                  frame condition #1 {
                    # "To prevent the Simple Error Handler VI from being loaded (e.g. when deploying to a Real-Time target), add the Conditional Disable Symbol \"DQMH_Disable_SEH\" to your project and set it to TRUE."
                  }
                }
                n178 = call-poly <vilib>:"Delacor_lib_QMH_Enqueue Message (poly).vi"("Priority Message? (F)"=TRUE, "Message"="Exit", "Message Queue in"=w353) -> ("error out"=w355:errorcluster)  [unwired: 7 in, 1 out]
              }
              frame True {
                # "If the module was launched externally, calling the Error Reported broadcast VI is the only action performed by the \"Error\" message. The module's caller can then process the error appropriately."
              }
            }
            n179 = Merge Errors(w348, w347) -> (w346:errorcluster)
          }
          frame "Simulate MHL Error" {
            # "#DQMH_HowTo The 'Simulate MHL Error' button  illustrates how the MHL handles errors. This event is instructional in nature and can be removed."
            # "Simulate an error occurring at the MHL"
            n180 = property on="Property Node" class="Mod Admin"(reference=w362) -> ("Accessors:Module ID"=w363:i32)  [unwired: 1 in, 2 out]
            n181 = call "Module Name--constant.vi"("Module ID"=w363) -> ("Module Name"=w358:string)  [unwired: 10 in]
            n182 = Format Into String(format string="Simulated error originating at Message Handling Loop in %s", w358) -> (resulting string=w359:string)  [unwired: 2 in, 1 out]
            n183 = call <vilib>:"Error Cluster From Error Code.vi"("show call chain? (False)"=TRUE, "error message (\"\")"=w359, "error code (0)"=5001) -> ("error out"=w365:errorcluster)  [unwired: 6 in]
            n184 = Merge Errors(w367, w365) -> (w366:errorcluster)
          }
          frame "Exit" {
            w378 = 91  # 91: not all Exit messages will have an argument
            w379 = TRUE  # Stop the VI
            # "Release the message queue reference"
            # "#CodeNeeded - Add any required cleanup code here."
            # "Exit - Exit the application."
            n185 = Variant To Data(error in=w386, type=T8 {"Module ID"=-1, "Origin"="", "Exit via Stop Module Req?"=FALSE, "Wait for Module to stop?"=FALSE} ("Stop Argument"), Variant=w377) -> (data=w374:T8, error out=w382:errorcluster)
            n186 = call <vilib>:"Clear Errors.vi"("error in (no error)"=w382, "specific error code to clear (0: all)"=w378) -> ("error out"=w385:errorcluster)  [unwired: 4 in, 1 out]
            n187 = property on="Property Node" class="Mod Admin"(reference=w372) -> ("Accessors:Module ID"=w371:i32)  [unwired: 1 in, 2 out]
            n188 = control-ref of="This VI"() -> (w373:refnum<vi>)
            n189 = call-dynamic "Delacor_lib_QMH_Release Message Queue.vi"("error in"=w385, "Message Queue"=w380) -> ("error out"=w384:errorcluster)  [unwired: 9 in]
            n190 = call "Handle Exit.vi"("Stop Argument"=w374, "Module Admin in"=w372, "VI reference"=w373) -> ("error out"=w383:errorcluster, "Wait for Stop?"=w375:bool)  [unwired: 7 in]
            n191 = Merge Errors(w384, w383) -> (w381:errorcluster)
            n192 = Unbundle By Name(w369) -> ("rSubPanel"=w368:refnum<vi>)
            n193 = call "Error Reported.vi"("Error"=w381, "Module ID"=w371) -> ()  [unwired: 9 in, 1 out]
            n194 = invoke class="SubPnl" method="Remove VI"(reference=w368) -> (error out=w370:errorcluster)  [unwired: 2 in, 2 out]
            n195 = call <vilib>:"Clear Errors.vi"("error in (no error)"=w370) -> ()  [unwired: 5 in, 2 out]
          }
          frame Default {
            # "'Default' case only runs if there is a message that isn't defined in any of the other cases.  Output a programming error."
            n196 = property on="Property Node" class="Mod Admin"(reference=w394) -> ("Accessors:Module ID"=w393:i32)  [unwired: 1 in, 2 out]
            n197 = call "Module Name--constant.vi"("Module ID"=w393) -> ("Module Name"=w387:string)  [unwired: 10 in]
            n198 = Format Into String(format string="The invalid message string \"%s\" was received in the Message Handling Loop for module \"%s\".", w388, w387) -> (resulting string=w390:string)  [unwired: 2 in, 1 out]
            n199 = call <vilib>:"Error Cluster From Error Code.vi"("show call chain? (False)"=TRUE, "error message (\"\")"=w390, "error code (0)"=1) -> ("error out"=w396:errorcluster)  [unwired: 6 in]
            n200 = Merge Errors(w397, w396) -> (w398:errorcluster)
          }
        }
        n201 = call-dynamic "Delacor_lib_QMH_Error Handler - Message Handling Loop.vi"("error in"=w198, "Message Queue in"=w189) -> ("dup error in"=w195:errorcluster)  [unwired: 8 in, 1 out]
      }
    }
    frame Error {
      n202 = call "Synchronize Caller Events.vi"("Module Admin"=w402) -> ("Module Admin out"=w401:refnum<class "Delacor_lib_QMH_Cloneable Module Admin.lvclass">)  [unwired: 9 in, 1 out]
      n203 = property on="Property Node" class="Mod Admin"(reference=w401) -> ("Accessors:Module ID"=w400:i32)  [unwired: 1 in, 2 out]
      n204 = call-dynamic "Delacor_lib_QMH_Release Message Queue.vi"("error in"=w408, "Message Queue"=w399) -> ("error out"=w407:errorcluster)  [unwired: 9 in]
      n205 = call "Module Name--constant.vi"("Module ID"=w400) -> ("Module Name"=w405:string)  [unwired: 10 in]
      n206 = Format Into String(format string="An error occurred during initialization. %s is no longer running.", w405) -> (resulting string=w403:string)  [unwired: 2 in, 1 out]
      n207 = call "Error Reported.vi"("Additional Information"=w403, "Error"=w407, "Module ID"=w400) -> ()  [unwired: 8 in, 1 out]
    }
  }
  n208 = Merge Errors(w19, w18) -> (w20:errorcluster)
  n209 = call "Close Module.vi"("error in"=w20, "Wait for stop?"=w4, "Module Admin in"=w6) -> ("error out"=w16:errorcluster, "External Launch"=w3:bool, "Module Admin out"=w5:refnum<class "Delacor_lib_QMH_Cloneable Module Admin.lvclass">)  [unwired: 6 in]
  n210 = Unregister For Events(event registration refnum=w11, error in=w16) -> (error out=w15:errorcluster)
  "error out" <- w15
  n211 = local write "Module Admin"(w5) -> ()
  n212 = case "External Launch?" shown="真" w3 {
    tunnel: w15 -> [_ w409]
    frame False {
    }
    frame True {
      n213 = case shown="无错误" w409 {
        frame No Error {
          n214 = invoke class="VI" method="FP.Close"() -> ()  [unwired: 3 in, 3 out]
        }
        frame Error {
          n215 = invoke class="VI" method="FP.Open"("Activate"=TRUE ("Activate?")) -> ()  [unwired: 4 in, 5 out]
        }
      }
    }
  }
